vi "Write UI References.vi"(8 "error in (no error)":errorcluster, 10 "UI References":T1, 11 "CIF_UI in":refnum<class "CIF_UI.lvclass">) -> (0 "error out":errorcluster, 3 "CIF_UI out":refnum<class "CIF_UI.lvclass">)   [LabVIEW 2021, in "CIF_UI.lvclass"]
uses:
  CIF_UI.lvclass
  Typedef/UI References.ctl
  Typedef/New Plugin.ctl
  Typedef/Channel Connection.ctl
  CIF_UI.lvclass/CIF_UI.ctl
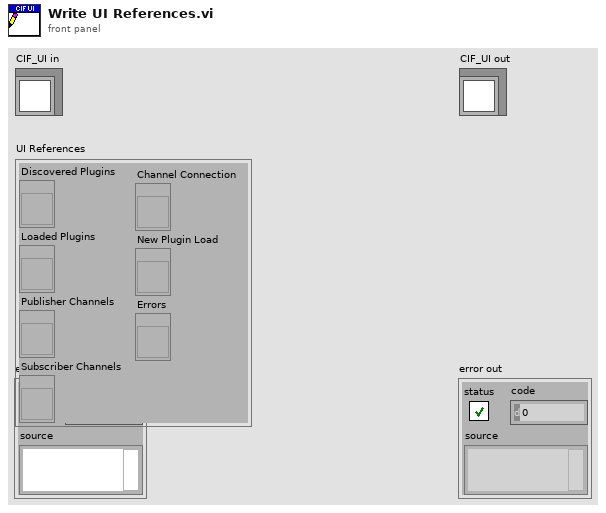
[diagram p1: front panel]
types:
  T1 = typedef "CIF_UI.lvclass/UI References.ctl" = cluster{"Discovered Plugins":refnum<vi>, "Loaded Plugins":refnum<vi>, "Publisher Channels":refnum<vi>, "Subscriber Channels":refnum<vi>, "New Plugin Load":refnum<vi>, "Errors":refnum<vi>, "Channel Connection":refnum<vi>}
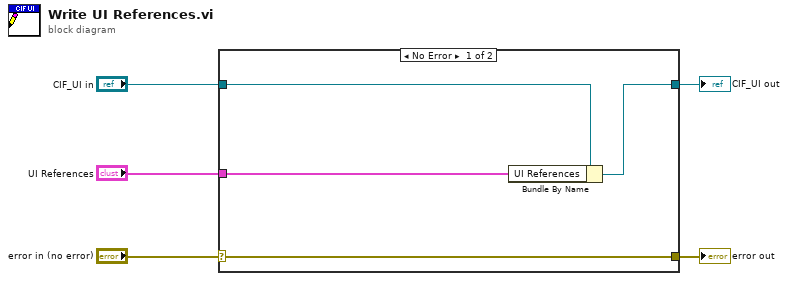
[diagram p0: block diagram]
diagram:
  n1 = case shown="No Error" "error in (no error)" {
    selector: "error in (no error)" -> [w9 w10]
    tunnel: [w9 w10] -> w4
    tunnel: [w7 w11] -> w2
    tunnel: "CIF_UI in" -> [w8 w11]
    tunnel: "UI References" -> [w6 _]
    frame No Error {
      n2 = Bundle By Name(cluster=w8, "UI References"=w6) -> (w7:refnum<class "CIF_UI.lvclass">)
    }
    frame Error {
    }
  }
  "error out" <- w4
  "CIF_UI out" <- w2
